vi "Read Samples (Complex DBL).vi"(8 "error in (no error)":errorcluster, 10 "Samples":i32, 11 "RTL-SDR in":refnum<class "Session.lvclass">) -> (0 "error out":errorcluster, 2 "Complex Array":cdb[](array[numeric]), 3 "RTL-SDR out":refnum<class "Session.lvclass">)   [LabVIEW 2021, in "RTL-SDR.lvlib" / "Session.lvclass"]
uses:
  Session.lvclass
  Session.lvclass/Session.ctl
  Read Bytes Sync.vi
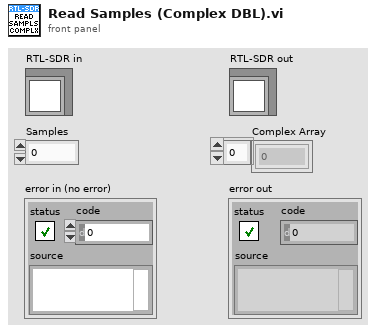
[diagram p1: front panel]
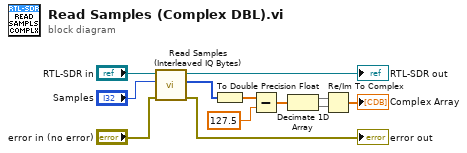
[diagram p0: block diagram]
diagram:
  n1 = call "Read Samples (Interleaved IQ Bytes).vi"("error in (no error)"="error in (no error)", "Samples"="Samples", "RTL-SDR in"="RTL-SDR in") -> ("error out"=→"error out":errorcluster, "Interleaved IQ Bytes"=w1:u8[], "RTL-SDR out"=→"RTL-SDR out":refnum<class "Session.lvclass">)  [unwired: 6 in]
  n2 = To Double Precision Float(number=w1) -> (double precision float=w10:dbl[])
  n3 = Subtract(x=w10, y=127.5) -> (x-y=w9:dbl[])
  n4 = Decimate 1D Array(w9) -> (w12:dbl[], w11:dbl[])
  n5 = Re/Im To Complex(1:w11, 2:w12) -> (0:→"Complex Array":cdb[])
